vi "PH_Trendviewer_Powermeter.panel.vi"(0 "object ref":refnum<vi>, 5 "error in (no error)":errorcluster) -> (19 "error out":errorcluster)   [LabVIEW 2014, in "PH_Trendviewer_Powermeter.lvlib"]
doc: "This is just an example for a GUI thread.\n\nLicense Agreement for this software:\n\nCopyright (C)\nGesellschaft für Schwerionenforschung, GSI\nPlanckstr. 1\n64291 Darmstadt\nGermany\n\nContact: D.Beck@gsi.de \n\nThis program is free software; you can redistribute it and/or modify it under the terms of the GNU General Public License as published by the Free Software Foundation; either version 2 of the license, or (at your option) any later version.\n\nThis program is distributed in the hope that it will be useful, but WITHOUT ANYW ARRANTY; without even the implied warranty of MERCHANTABILITY or FITNESS FOR A PARTICULAR PURPOSE. See the GNU General License for more details (http://www.gnu.org).\n\nGesellschaft für Schwerionenforschung, GSI\nPlanckstr. 1, 64291 Darmstadt, Germany\nFor all questions and ideas contact: M.Richter@gsi.de, H.Brand@gsi.de or D.Beck@gsi.de.\nLast update: 18-DEC-2002"
uses:
  PH_Trendviewer_Powermeter.lvlib
  PH_Basics/PH_Common/PH_Common.lvlib
  CS_Core/CSSystem/CSSystemLib/CSSystemLib.lvlib
  PH_Basics/PH_Class/PH_Class.lvlib
panel:
  in  "Start":bool
  in  "Stat or Trend":bool
  in  "Export Data":bool
  out "Result Graph":cluster{dbl[], dbl[]}[](graph)
  in  "Dummy Std Dev":string caption="Std Dev"
  in  "Dummy Mean":string caption="Mean"
  out "Std Dev Data":dbl caption="Unit" format="%#_4p"
  out "Mean Data":dbl caption="Unit" format="%#_4p"
  out "Status":u32(colorbox)
  in  "Operator":string
  in  "Delete":bool
  # "PCS"
  # "3.40"
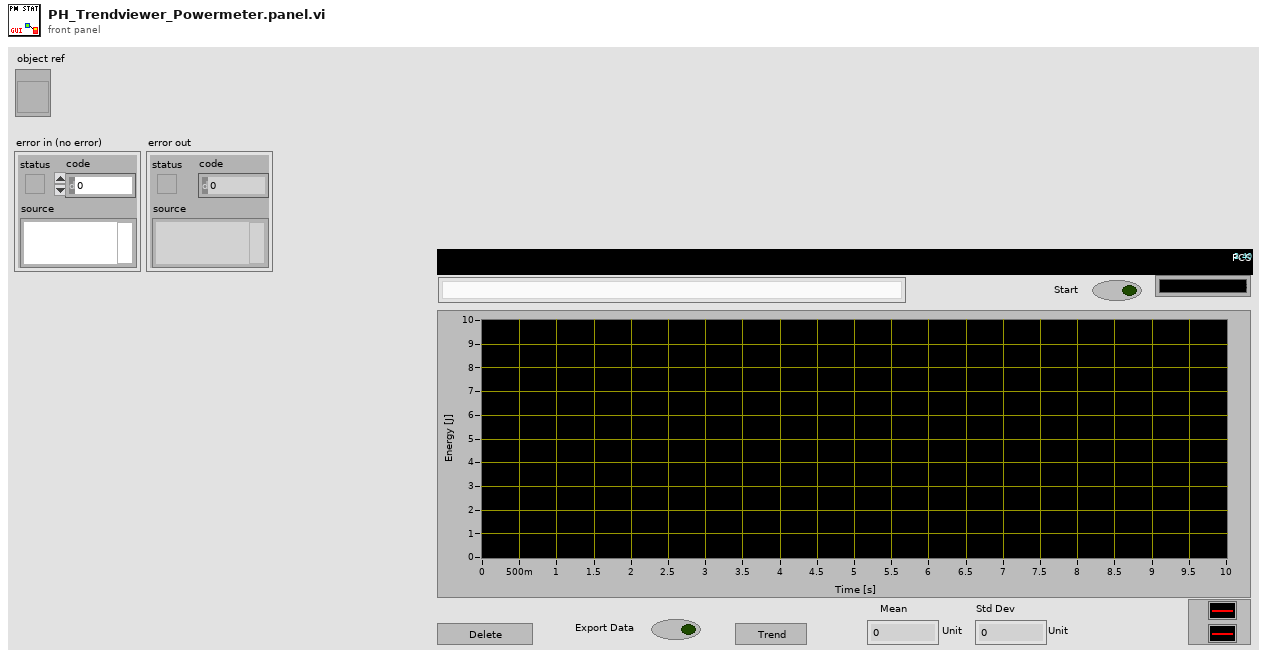
[diagram p1: front panel]
types:
  T1 = enum8{"Enabled", "Disabled", "Disabled and Grayed Out"}
  T2 = typedef "PH_Trendviewer_Powermeter.lvlib/PH_Trendviewer_Powermeter.i attribute.ctl" = cluster{"GUI Refs ":cluster{"Status":refnum<vi>, "Result Graph":refnum<vi>, "Mean Data":refnum<vi>, "Std Dev Data":refnum<vi>, "Dummy Mean":refnum<vi>, "Dummy Std Dev":refnum<vi>, "Export Data":refnum<vi>, "Stat or Trend":refnum<vi>, "Delete":refnum<vi>, "Powermeter":refnum<vi>, "Start":refnum<vi>}, "Powermeter":string, "Stat or Trend":bool, "Start":bool, "Data":cluster{"Time Stamp":timestamp, "Energy [J]":dbl}[], "Datasets strored":i32, "Dataarray Size":i32}
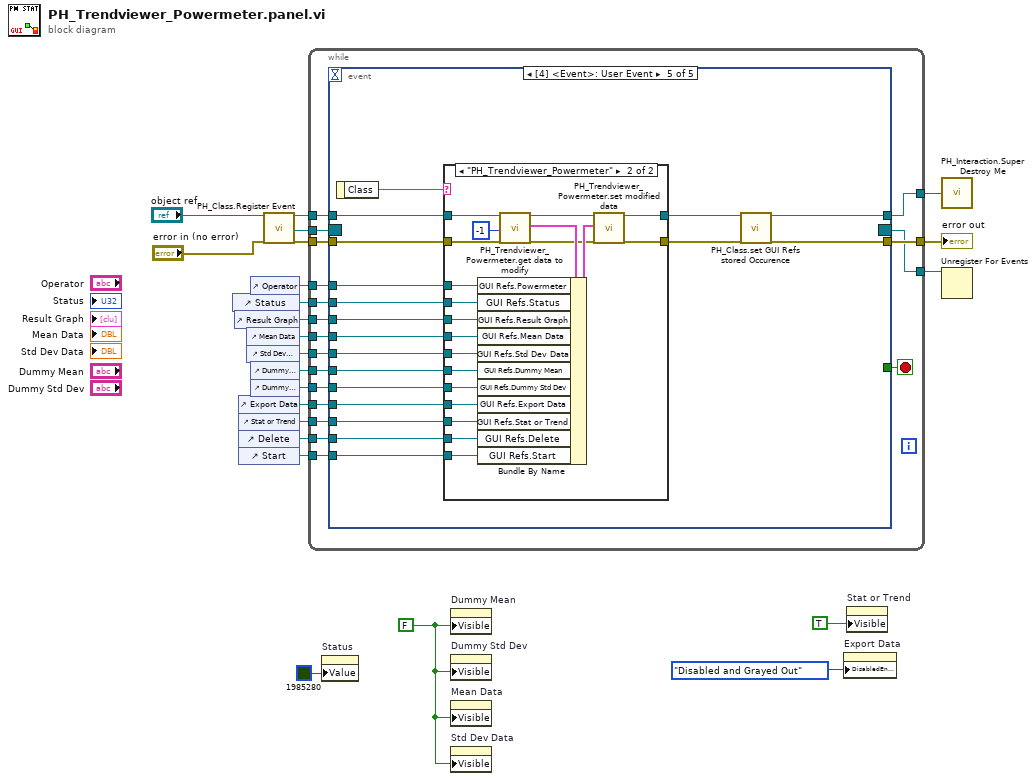
[diagram p0: block diagram]
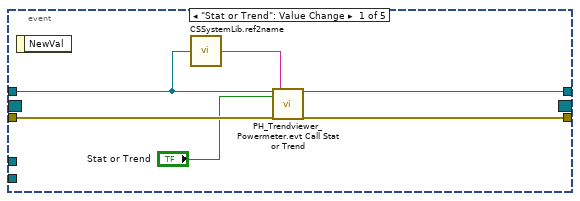
[diagram p2: hidden frame]
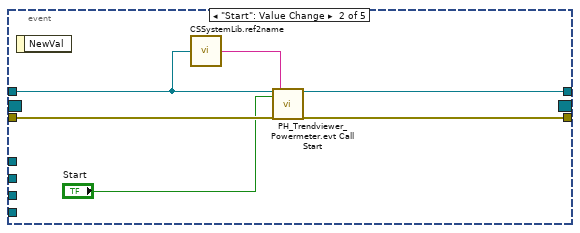
[diagram p3: hidden frame]
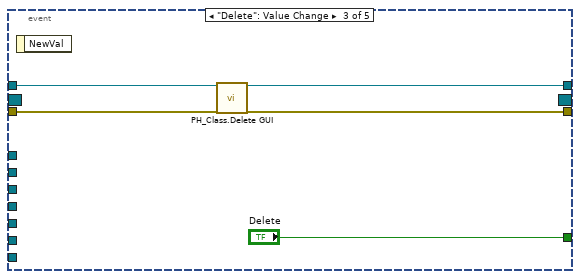
[diagram p4: hidden frame]
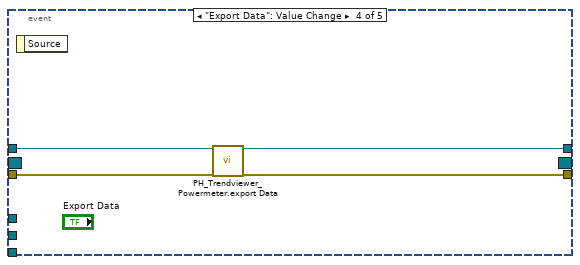
[diagram p5: hidden frame]
diagram:
  w21 = FALSE
  n1 = control-ref of="Status"() -> (w10:refnum<vi>)
  n2 = control-ref of="Result Graph"() -> (w9:refnum<vi>)
  n3 = control-ref of="Export Data"() -> (w4:refnum<vi>)
  n4 = control-ref of="Stat or Trend"() -> (w3:refnum<vi>)
  n5 = control-ref of="Delete"() -> (w2:refnum<vi>)
  n6 = control-ref of="Start"() -> (w1:refnum<vi>)
  n7 = control-ref of="Mean Data"() -> (w8:refnum<vi>)
  n8 = control-ref of="Std Dev Data"() -> (w7:refnum<vi>)
  n9 = control-ref of="Operator"() -> (w11:refnum<vi>)
  n10 = control-ref of="Dummy Mean"() -> (w6:refnum<vi>)
  n11 = control-ref of="Dummy Std Dev"() -> (w5:refnum<vi>)
  n12 = call "PH_Class.Register Event.vi"("i ref in"="object ref", "error in (no error)"="error in (no error)") -> ("i ref out"=w17:refnum<vi>, "Event Registration Refnum"=w15:refnum<event-registration>, "error out"=w16:errorcluster)  [unwired: 15 in]
  n13 = while {
    tunnel: [w40] -> w23
    tunnel: [w39] -> w22
    tunnel: w17 -> [w38]
    tunnel: w16 -> [w37]
    tunnel: w15 -> [w36]
    tunnel: [w35] -> w14
    tunnel: w11 -> [w34]
    tunnel: w10 -> [w33]
    tunnel: w9 -> [w32]
    tunnel: w8 -> [w31]
    tunnel: w7 -> [w30]
    tunnel: w6 -> [w29]
    tunnel: w5 -> [w28]
    tunnel: w4 -> [w27]
    tunnel: w3 -> [w26]
    tunnel: w2 -> [w25]
    tunnel: w1 -> [w24]
    stop <- w41 stop-if-true
    n14 = event shown="[4] <Event>: User Event" {
      selector: w36 -> [_ _ _ _ _]
      dyn-events: [_ _ _ _ _] -> w35
      timeout: _ -> [_ _ _ _ _]
      tunnel: [_ _ "Delete" _ _] -> w41
      tunnel: w38 -> [w43 w49 w57 w61 w80]
      tunnel: [w45 w51 w56 w59 w78] -> w40
      tunnel: [w46 w52 w54 w60 w75] -> w39
      tunnel: w37 -> [w47 w53 w55 w62 w77]
      tunnel: w34 -> [_ _ _ _ w73]
      tunnel: w33 -> [_ _ _ _ w72]
      tunnel: w32 -> [_ _ _ _ w71]
      tunnel: w31 -> [_ _ _ _ w70]
      tunnel: w30 -> [_ _ _ _ w69]
      tunnel: w29 -> [_ _ _ _ w68]
      tunnel: w28 -> [_ _ _ _ w67]
      tunnel: w27 -> [_ _ _ _ w66]
      tunnel: w26 -> [_ _ _ _ w65]
      tunnel: w25 -> [_ _ _ _ w64]
      tunnel: w24 -> [_ _ _ _ w63]
      event "Stat or Trend": Value Change {
        n15 = event-data() -> ()  [unwired: 1 in, 1 out]
        n16 = call "CSSystemLib.ref2name.vi"("obj refnum"=w43) -> ("name"=w44:string)
        n17 = call "PH_Trendviewer_Powermeter.evt Call Stat or Trend.vi"("i ref in"=w43, "Stat or Trend"="Stat or Trend", "error in (no error)"=w47, "Instance"=w44) -> ("i ref out"=w45:refnum<vi>, "error out"=w46:errorcluster)  [unwired: 14 in]
      }
      event "Start": Value Change {
        n18 = event-data() -> ()  [unwired: 1 in, 1 out]
        n19 = call "CSSystemLib.ref2name.vi"("obj refnum"=w49) -> ("name"=w50:string)
        n20 = call "PH_Trendviewer_Powermeter.evt Call Start.vi"("i ref in"=w49, "Start"="Start", "error in (no error)"=w53, "Instance"=w50) -> ("i ref out"=w51:refnum<vi>, "error out"=w52:errorcluster)  [unwired: 14 in]
      }
      event "Delete": Value Change {
        n21 = event-data() -> ()  [unwired: 1 in, 1 out]
        n22 = call "PH_Class.Delete GUI.vi"("VI in"=w57, "error in (no error)"=w55) -> ("VI out"=w56:refnum<vi>, "error out"=w54:errorcluster)  [unwired: 16 in]
      }
      event "Export Data": Value Change {
        n23 = event-data() -> ()  [unwired: 1 in, 1 out]
        n24 = call "PH_Trendviewer_Powermeter.export Data.vi"("i ref in"=w61, "error in (no error)"=w62) -> ("i ref out"=w59:refnum<vi>, "error out"=w60:errorcluster)  [unwired: 16 in]
      }
      event User Event {
        n25 = event-data() -> ("Class"=w74:string)  [unwired: 1 in]
        n26 = case shown="\"PH_Trendviewer_Powermeter\"" w74 {
          tunnel: w80 -> [w82 w99]
          tunnel: [w82 w97] -> w79
          tunnel: w77 -> [w81 w96]
          tunnel: [w81 w94] -> w76
          tunnel: w73 -> [_ w93]
          tunnel: w72 -> [_ w92]
          tunnel: w71 -> [_ w91]
          tunnel: w70 -> [_ w90]
          tunnel: w69 -> [_ w89]
          tunnel: w68 -> [_ w88]
          tunnel: w67 -> [_ w87]
          tunnel: w66 -> [_ w86]
          tunnel: w65 -> [_ w85]
          tunnel: w64 -> [_ w84]
          tunnel: w63 -> [_ w83]
          frame Default {
          }
          frame "PH_Trendviewer_Powermeter" {
            n27 = call "PH_Trendviewer_Powermeter.get data to modify.vi"("i ref in"=w99, "ms timeout (10000)"=-1, "error in (no error)"=w96) -> ("i ref out"=w98:refnum<vi>, "i attribute"=w101:T2, "error out"=w95:errorcluster)  [unwired: 13 in, 1 out]
            n28 = Bundle By Name(cluster=w101, "GUI Refs.Powermeter"=w93, "GUI Refs.Status"=w92, "GUI Refs.Result Graph"=w91, "GUI Refs.Mean Data"=w90, "GUI Refs.Std Dev Data"=w89, "GUI Refs.Dummy Mean"=w88, "GUI Refs.Dummy Std Dev"=w87, "GUI Refs.Export Data"=w86, "GUI Refs.Stat or Trend"=w85, "GUI Refs.Delete"=w84, "GUI Refs.Start"=w83) -> (w100:T2)
            n29 = call "PH_Trendviewer_Powermeter.set modified data.vi"("i ref in"=w98, "i attribute"=w100, "error in (no error)"=w95) -> ("i ref out"=w97:refnum<vi>, "error out"=w94:errorcluster)  [unwired: 15 in]
          }
        }
        n30 = call "PH_Class.set GUI Refs stored Occurence.vi"("i ref in"=w79, "error in (no error)"=w76) -> ("i ref out"=w78:refnum<vi>, "error out"=w75:errorcluster)  [unwired: 16 in]
      }
    }
  }
  "error out" <- w22
  n31 = property on="Status" class="ColBox"("Value"=u32 1985280 ("Status")) -> ()  [unwired: 2 in, 2 out]
  n32 = property on="Dummy Mean" class="Str"("Visible"=w21) -> ()  [unwired: 2 in, 2 out]
  n33 = property on="Dummy Std Dev" class="Str"("Visible"=w21) -> ()  [unwired: 2 in, 2 out]
  n34 = property on="Mean Data" class="DigNum (strict)"("Visible"=w21) -> ()  [unwired: 2 in, 2 out]
  n35 = property on="Std Dev Data" class="DigNum (strict)"("Visible"=w21) -> ()  [unwired: 2 in, 2 out]
  n36 = property on="Export Data" class="Bool"("DisabledEnum"=T1."Disabled and Grayed Out" ("Disabled")) -> ()  [unwired: 2 in, 2 out]
  n37 = property on="Stat or Trend" class="Bool (strict)"("Visible"=TRUE) -> ()  [unwired: 2 in, 2 out]
  n38 = call "PH_Interaction.Super Destroy Me.vi"("i ref out"=w23) -> ()
  n39 = Unregister For Events(event registration refnum=w14) -> ()  [unwired: 1 in, 1 out]
